vi "setFreqData.vi"(2 "error in (no error)":errorcluster, 3 "String":string, 4 "FrequencyCounter.lvclass":refnum<class "FrequencyCounter.lvclass">) -> (0 "error out":errorcluster, 1 "FrequencyCounter.lvclass 2":refnum<class "FrequencyCounter.lvclass">)   [LabVIEW 2011, in "Hardware.lvlib" / "frequencyCounters.lvlib" / "FrequencyCounter.lvclass"]
uses:
  FrequencyCounter.lvclass
  FrequencyCounter.lvclass/FrequencyCounter.ctl
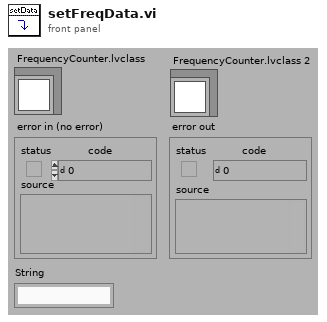
[diagram p1: front panel]
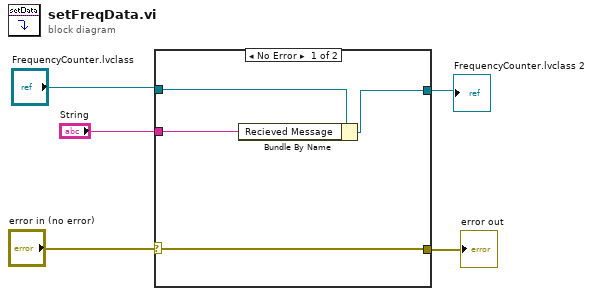
[diagram p0: block diagram]
diagram:
  n1 = case shown="No Error" "error in (no error)" {
    selector: "error in (no error)" -> [w7 w11]
    tunnel: [w7 w11] -> w4
    tunnel: "FrequencyCounter.lvclass" -> [w9 w10]
    tunnel: [w8 w10] -> w2
    tunnel: "String" -> [w6 _]
    frame No Error {
      n2 = Bundle By Name(cluster=w9, "Recieved Message"=w6) -> (w8:refnum<class "FrequencyCounter.lvclass">)
    }
    frame Error {
    }
  }
  "error out" <- w4
  "FrequencyCounter.lvclass 2" <- w2
